vi "Configure Ranges.vi"(8 "error in (no error)":errorcluster, 10 "ranges":u16[](array[ring]) items=["0.01 mbar", "0.01 Torr", "0.02 mbar", "0.02 Torr", "0.05 mbar", "0.05 Torr", "0.1 mbar", "0.1 Torr", "0.25 mbar", "0.25 Torr", "0.5 mbar", "0.5 Torr", "1 mbar", "1 Torr", "2 mbar", "2 Torr", "5 mbar", "5 Torr", "10 mbar", "10 Torr", "20 mbar", "20 Torr", "50 mbar", "50 Torr", "100 mbar", "100 Torr", "200 mbar", "200 Torr", "500 mbar", "500 Torr", "1000 mbar", "1100 mbar", "1000 Torr", "2 bar", "5 bar", "10 bar", "50 bar"], 11 "VGC in":refnum<class "PL Inficon VGC.lvclass">) -> (0 "error out":errorcluster, 2 "ranges":u16[](array[ring]) items=["0.01 mbar", "0.01 Torr", "0.02 mbar", "0.02 Torr", "0.05 mbar", "0.05 Torr", "0.1 mbar", "0.1 Torr", "0.25 mbar", "0.25 Torr", "0.5 mbar", "0.5 Torr", "1 mbar", "1 Torr", "2 mbar", "2 Torr", "5 mbar", "5 Torr", "10 mbar", "10 Torr", "20 mbar", "20 Torr", "50 mbar", "50 Torr", "100 mbar", "100 Torr", "200 mbar", "200 Torr", "500 mbar", "500 Torr", "1000 mbar", "1100 mbar", "1000 Torr", "2 bar", "5 bar", "10 bar", "50 bar"], 3 "VGC out":refnum<class "PL Inficon VGC.lvclass">)   [LabVIEW 2015, in "PL Inficon VGC.lvclass"]
doc: "Configures full scale measurement ranges."
uses:
  PL Inficon VGC.lvclass
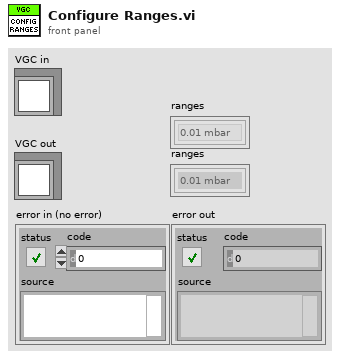
[diagram p1: front panel]
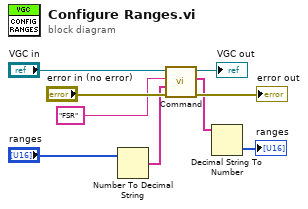
[diagram p0: block diagram]
diagram:
  n1 = Number To Decimal String(number="ranges") -> (decimal integer string=w1:string[])  [unwired: 1 in]
  n2 = call "Command.vi"("error in (no error)"="error in (no error)", "parameters"=w1, "command"="FSR" ("format string"), "VGC in"="VGC in") -> ("error out"=→"error out":errorcluster, "response data"=w5:string[], "VGC out"=→"VGC out":refnum<class "PL Inficon VGC.lvclass">)  [unwired: 5 in]
  n3 = Decimal String To Number(string=w5) -> (number=→"ranges":i32[])  [unwired: 2 in, 1 out]
